vi "tsapp_connect.vi"(8 "error in (no error)":errorcluster, 11 "Path":path) -> (0 "error out":errorcluster, 2 "retuen":i32, 3 "Path output":path)   [LabVIEW 2014]
doc: "Function Introduction ：\nConnect the application. When this function is executed, it will check whether all mapped hardware channels are complete\nReady, set various hardware parameters, and complete the connection between the device and the application program.\nCall location ：\nAfter setting the hardware parameters, call this function to complete the connection of the device. behind\nYou can call the device to complete functions such as data transmission and reception.\ninput parameter ：\nnothing\nReturn value ：\n==0: Connection successful\nOther, query error codes"
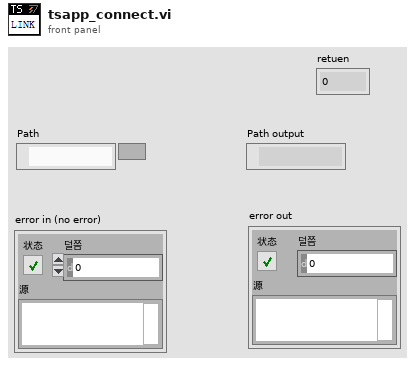
[diagram p1: front panel]
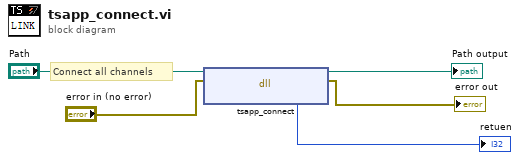
[diagram p0: block diagram]
diagram:
  # "Connect all channels"
  n1 = dll-call lib="PTH2Habs CUsers\nAdministratorDesktopTS_Can通讯PathTSMaster.dll" fn="tsapp_connect"(path in="Path", error in="error in (no error)") -> (path out=→"Path output":path, error out=→"error out":errorcluster, "tsapp_connect"=→"retuen":i32)  [unwired: 1 in]
